vi "Test Filt.vi"() -> ()   [LabVIEW 2024, in "Spectrum Recorder too.lvclass"]
uses:
  Spectrum Recorder too.lvclass
  NHMFL_Core/Libraries/Red Pitaya/RP Core/Red Pitaya Transceiver Driver/Red Pitaya Transceiver Driver.lvclass
  Spectrum Recorder too.lvclass/Spectrum Recorder too.ctl
  NHMFL_Core/Libraries/Red Pitaya/RP Core/RP Transceiver/RP Transceiver.lvclass
  NHMFL_Core/Libraries/Instruments/Instrument Driver/Instrument Driver.lvclass
  NHMFL_Core/Libraries/Instruments/Instrument Driver/Worker State.ctl
  NHMFL_Core/Libraries/Red Pitaya/RP Core/Red Pitaya Transceiver Driver/Spectrum Configuration.ctl
panel:
  out "Status response":u32=1 format="0x%x (%d)"
  out "Waveform Graph":i32[][](graph)
  in  "N point out":i32=16384 format="0x%x (%d)"
  out "Pre -data out 2":i32[](array[numeric])
  out "Pre-data out":i32[](array[numeric])
  out "Points in buffer init":i32
  out "y counter init":u32=1 format="0x%x (%d)"
  out "f counter init":u32=1 format="0x%x (%d)"
  in  "Counters":i32[][](array[numeric])
  in  "Pre-trigger samples":u64
  in  "Post-trigger samples":u64=33554432 format="%.0f (x%x)"
  out "y counter 2":u32=2999 format="0x%x (%d)"
  out "Points in buffer 2":i32=3000
  out "f counter 2":u32=2998 format="0x%x (%d)"
  out "Points in buffer":i32=3003
  out "f counter":u32=3001 format="0x%x (%d)"
  out "y counter":u32=3002 format="0x%x (%d)"
  in  "milliseconds to wait":u32=5000
  out "size(s)":i32=3003
  out "Y":i32[](array[numeric])
  out "X":i32[](array[numeric])
  out "F":dbl[](array[numeric]) format="%_6p"
  out "Sweep duration":dbl=0.786694144 format="%#_gs"
  in  "Configuration":T1={"Start frequency"=500000.0, "End frequency"=2000000.0, "Coarse step"=10000.0, "Step duration"=6.5536e-05, "Red Pitaya address"="192.168.1.120", "Open plot \non start"=TRUE, "Regions width"=2000.0, "Fine step"=10.0, "Pause between scans"=1.0, "Clear rgs on start"=FALSE, "Output amplitude"=1.0, "Append measurements"=[], "Full scan period"=nan, "Full start"=500000.0, "Full end"=2000000.0, "Full step"=100.0} {"Full step" format="%#_6pHz"; "Full end" format="%#_6pHz"; "Full start" format="%#_6pHz"; "Full scan period" format="%#_6fs"; "Output amplitude" min=0.0 max=1.0 step=0.1 format="%#_6pV"; "Pause between scans" format="%#_6ps"; "Fine step" min=0.001 format="%#_6pHz"; "Regions width" format="%#_6pHz"; "Step duration" format="%#_6ps"; "Coarse step" format="%#_6pHz"; "End frequency" format="%#_6pHz"; "Start frequency" format="%#_6pHz"}
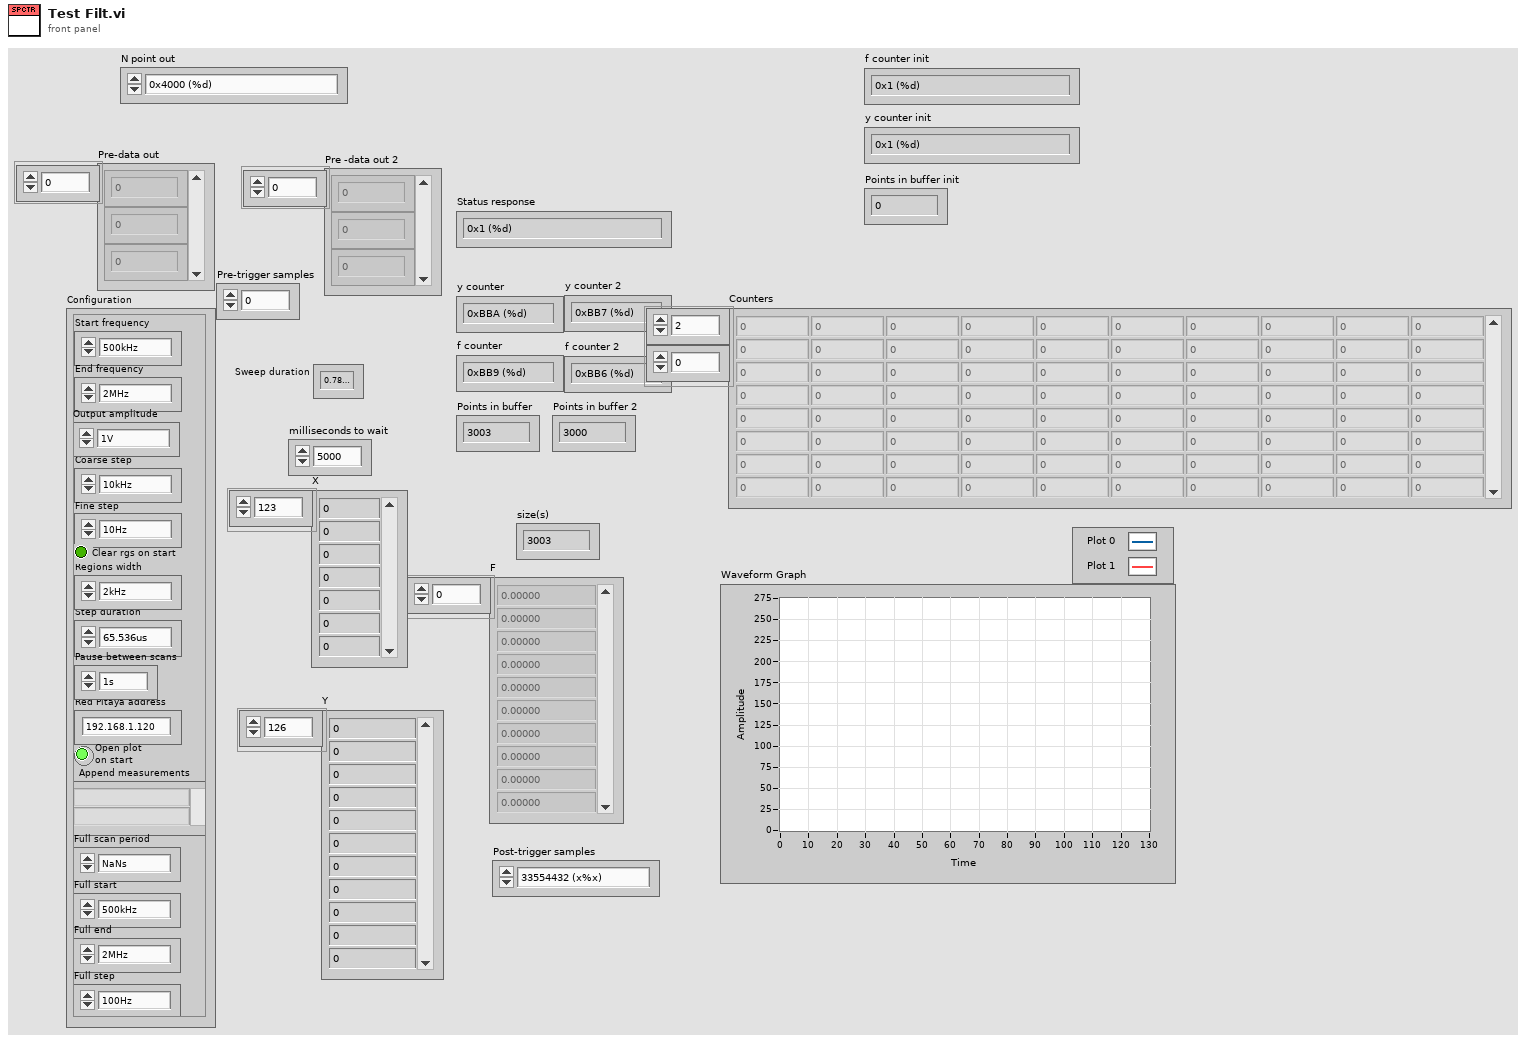
[diagram p1: front panel]
types:
  T1 = typedef "Spectrum Configuration.ctl" = cluster{"Start frequency":dbl, "End frequency":dbl, "Coarse step":dbl, "Step duration":dbl, "Red Pitaya address":string, "Open plot \non start":bool, "Regions width":dbl, "Fine step":dbl, "Pause between scans":dbl, "Clear rgs on start":bool, "Output amplitude":dbl, "Append measurements":string[], "Full scan period":dbl, "Full start":dbl, "Full end":dbl, "Full step":dbl}
  T2 = typedef "Worker State.ctl" = enum16{"Idle", "Starting", "Working", "Stopping"}
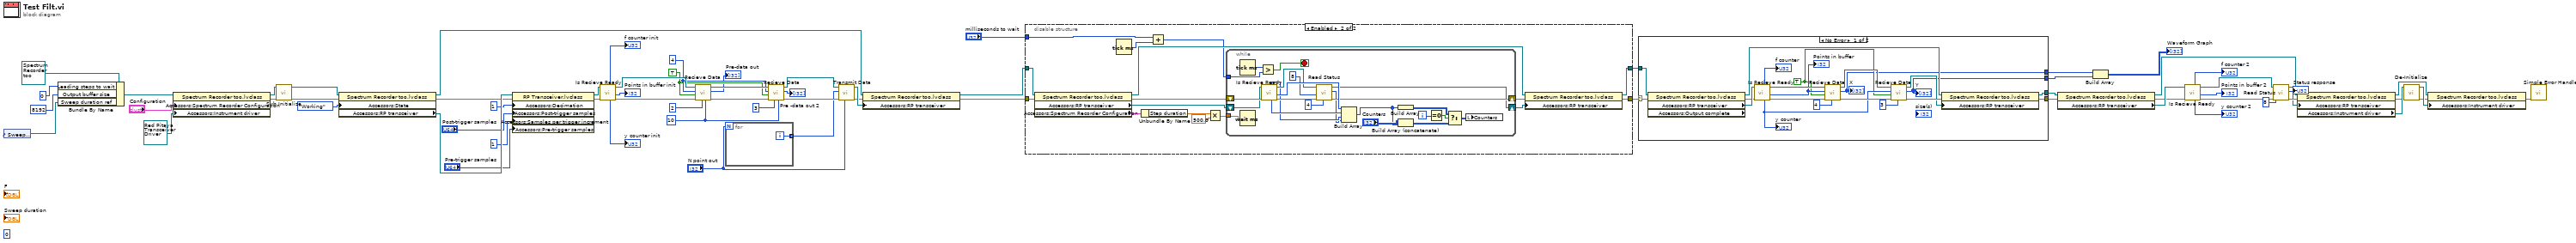
[diagram p0: block diagram]
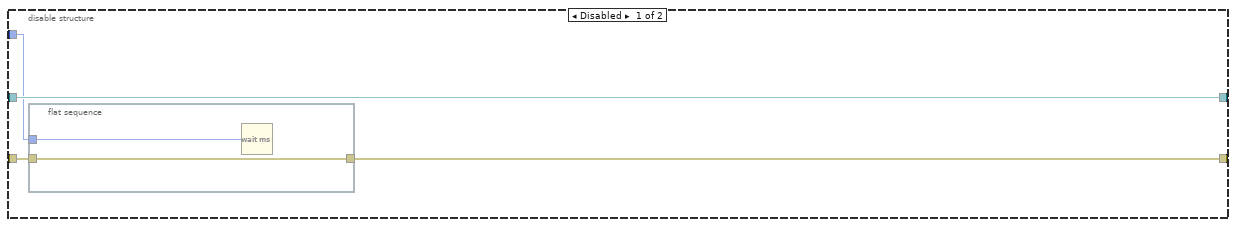
[diagram p2: hidden frame]
diagram:
  w22 = 10 ("timeout ms (25000)")
  w25 = u32 4 ("Points to read")
  w24 = TRUE ("Force read")
  (unwired) i16 0
  n1 = control-ref of="Sweep duration"() -> (w62:refnum<vi>)
  n2 = Bundle By Name(cluster=refnum<class "Spectrum Recorder too.lvclass"> refnum ("Spectrum Recorder too.lvclass"), "Leading steps to wait"=0, "Output buffer size"=8192, "Sweep duration ref"=w62) -> (w63:refnum<class "Spectrum Recorder too.lvclass">)
  n3 = property class="Spectrum Recorder too.lvclass"(reference=w63, "Accessors:Spectrum Recorder Configuration"="Configuration", "Accessors:Instrument driver"=refnum<class "Red Pitaya Transceiver Driver.lvclass"> refnum ("Red Pitaya Transceiver Driver.lvclass")) -> (reference out=w67:refnum<class "Spectrum Recorder too.lvclass">, error out=w65:errorcluster)  [unwired: 1 in]
  n4 = call-dynamic "Sub Initialize.vi"("error in (no error)"=w65, "Spectrum Recorder in"=w67) -> ("error out"=w66:errorcluster, "Spectrum Recorder out"=w58:refnum<class "Spectrum Recorder too.lvclass">)  [unwired: 7 in, 1 out]
  n5 = property class="Spectrum Recorder too.lvclass"(reference=w58, error in=w66, "Accessors:State"=Worker_State."Working" ("State")) -> (reference out=w31:refnum<class "Spectrum Recorder too.lvclass">, error out=w49:errorcluster, "Accessors:RP transceiver"=w52:refnum<class "RP Transceiver.lvclass">)
  n6 = property class="RP Transceiver.lvclass"(reference=w52, error in=w49, "Accessors:Decimation"=1 ("Decimation"), "Accessors:Post-trigger samples"="Post-trigger samples", "Accessors:Samples per trigger increment "=1 ("Samples per trigger increment"), "Accessors:Pre-trigger samples"="Pre-trigger samples") -> (reference out=w19:refnum<class "RP Transceiver.lvclass">, error out=w18:errorcluster)
  n7 = call-dynamic "Is Recieve Ready.vi"("error in (no error)"=w18, "RP Instrument in"=w19) -> ("error out"=w26:errorcluster, "Points in buffer"=→"Points in buffer init":u32, "RP Instrument out"=w29:refnum<class "RP Transceiver.lvclass">, "y counter"=→"y counter init":u32, "f counter"=→"f counter init":u32)  [unwired: 4 in, 1 out]
  n8 = call-dynamic "Recieve Data.vi"("timeout ms (25000)"=w22, "hub port"=u64 2, "error in (no error)"=w26, "Force read"=w24, "Points to read"=w25, "RP Instrument in"=w29) -> ("error out"=w27:errorcluster, "Data out"=→"Pre-data out":i32[], "RP Instrument out"=w28:refnum<class "RP Transceiver.lvclass">)  [unwired: 3 in]
  n9 = for {
    N: "N point out" -> [_]
    tunnel: [w70] -> w13 mode=indexing
    i -> [w70]
  }
  n10 = call-dynamic "Recieve Data.vi"("timeout ms (25000)"=w22, "hub port"=u64 3, "error in (no error)"=w27, "Force read"=w24, "Points to read"=w25, "RP Instrument in"=w28) -> ("error out"=w15:errorcluster, "Data out"=→"Pre -data out 2":i32[], "RP Instrument out"=w17:refnum<class "RP Transceiver.lvclass">)  [unwired: 3 in]
  n11 = call-dynamic "Transmit Data.vi"("Buffer size"="N point out", "error in (no error)"=w15, "Data"=w13, "RP Instrument in"=w17) -> ("error out"=w14:errorcluster, "RP Instrument out"=w16:refnum<class "RP Transceiver.lvclass">)  [unwired: 6 in]
  n12 = property class="Spectrum Recorder too.lvclass"(reference=w31, error in=w14, "Accessors:RP transceiver"=w16) -> (reference out=w42:refnum<class "Spectrum Recorder too.lvclass">, error out=w56:errorcluster)
  n13 = disable-structure shown="Enabled" {
    disable-tunnel: w56 -> [w74 w92]
    disable-tunnel: [w73 w88] -> w55
    disable-tunnel: w42 -> [w72 w85]
    disable-tunnel: [w72 w87] -> w41
    disable-tunnel: "milliseconds to wait" -> [w71 w78]
    frame Disabled {
      n14 = flat-sequence {
        tunnel: w74 -> [w76]
        tunnel: [w76] -> w73
        tunnel: w71 -> [w75]
        frame #0 {
          n15 = Wait (ms)(milliseconds to wait=w75) -> ()  [unwired: 1 out]
        }
      }
    }
    frame Enabled {
      n16 = property class="Spectrum Recorder too.lvclass"(reference=w85, error in=w92) -> (reference out=w86:refnum<class "Spectrum Recorder too.lvclass">, error out=w84:errorcluster, "Accessors:RP transceiver"=w91:refnum<class "RP Transceiver.lvclass">, "Accessors:Spectrum Recorder Configuration"=w83:T1)
      n17 = Tick Count (ms)() -> (millisecond timer value=w79:u32)
      n18 = Unbundle By Name(w83) -> ("Step duration"=w82:dbl)
      n19 = Add(x=w78, y=w79) -> (x+y=w77:u32)
      n20 = Multiply(x=w82, y=500.0) -> (x*y=w80:dbl)
      n21 = while {
        shift-right: [w97] -> w90
        shift-left: w84 -> [w115]
        shift-right: [w96] -> w89
        shift-left: w91 -> [w114]
        tunnel: w80 -> [w113]
        tunnel: w77 -> [w101]
        i -> [w111]
        stop <- w112 stop-if-true
        n22 = Tick Count (ms)() -> (millisecond timer value=w102:u32)
        n23 = Wait (ms)(milliseconds to wait=w113) -> ()  [unwired: 1 out]
        n24 = Greater?(x=w102, y=w101) -> (0:w112:bool)
        n25 = call-dynamic "Is Recieve Ready.vi"("error in (no error)"=w115, "RP Instrument in"=w114) -> ("error out"=w99:errorcluster, "Points in buffer"=w110:u32, "RP Instrument out"=w100:refnum<class "RP Transceiver.lvclass">, "y counter"=w109:u32, "f counter"=w94:u32)  [unwired: 4 in, 1 out]
        n26 = call-dynamic "Read Status.vi"("bytes to read"=4, "error in (no error)"=w99, "Status offset"=u64 8, "RP Instrument in"=w100) -> ("error out"=w97:errorcluster, "Status response"=w93:u32, "RP Instrument out"=w96:refnum<class "RP Transceiver.lvclass">)  [unwired: 5 in]
        n27 = Build Array(w110, w109, w94, w93) -> (w105:u32[])
        n28 = Build Array(w105) -> (w107:u32[][])
        n29 = Build Array (concatenate)("Counters", w105) -> (w104:u32[][])
        n30 = Equal To 0?(x=w111) -> (x = 0?=w108:bool)
        n31 = Select(t=w107, s=w108, f=w104) -> (s? t:f=w103:u32[][])
        n32 = local write "Counters"(w103) -> ()
      }
      n33 = property class="Spectrum Recorder too.lvclass"(reference=w86, error in=w90, "Accessors:RP transceiver"=w89) -> (reference out=w87:refnum<class "Spectrum Recorder too.lvclass">, error out=w88:errorcluster)
    }
  }
  n34 = case shown="No Error" w55 {
    selector: w55 -> [w135 w137]
    tunnel: [w136 w137] -> w48
    tunnel: [w130 w138] -> w33
    tunnel: w41 -> [w134 w138]
    tunnel: [w117 _] -> w11
    tunnel: [w116 _] -> w10
    frame No Error {
      w118 = TRUE ("Force read")
      n35 = property class="Spectrum Recorder too.lvclass" props=["Accessors:RP transceiver", "Accessors:Output complete"](reference=w134, error in=w135) -> (reference out=w131:refnum<class "Spectrum Recorder too.lvclass">, error out=w132:errorcluster, "Accessors:RP transceiver"=w133:refnum<class "RP Transceiver.lvclass">)  [unwired: 1 out]
      n36 = call-dynamic "Is Recieve Ready.vi"("error in (no error)"=w132, "RP Instrument in"=w133) -> ("error out"=w125:errorcluster, "Points in buffer"=w121:u32, "RP Instrument out"=w124:refnum<class "RP Transceiver.lvclass">, "y counter"=w120:u32, "f counter"=→"f counter":u32)  [unwired: 4 in, 1 out]
      "y counter" <- w120
      "Points in buffer" <- w121
      n37 = call-dynamic "Recieve Data.vi"("hub port"=u64 4, "error in (no error)"=w125, "Force read"=w118, "Points to read"=w121, "RP Instrument in"=w124) -> ("error out"=w127:errorcluster, "Data out"=w117:i32[], "RP Instrument out"=w126:refnum<class "RP Transceiver.lvclass">)  [unwired: 4 in]
      "X" <- w117
      n38 = call-dynamic "Recieve Data.vi"("hub port"=u64 3, "error in (no error)"=w127, "Force read"=w118, "Points to read"=w120, "RP Instrument in"=w126) -> ("error out"=w123:errorcluster, "Data out"=w116:i32[], "RP Instrument out"=w122:refnum<class "RP Transceiver.lvclass">)  [unwired: 4 in]
      "Y" <- w116
      n39 = property class="Spectrum Recorder too.lvclass"(reference=w131, error in=w123, "Accessors:RP transceiver"=w122) -> (reference out=w130:refnum<class "Spectrum Recorder too.lvclass">, error out=w136:errorcluster)
    }
    frame Error {
    }
  }
  n40 = property class="Spectrum Recorder too.lvclass"(reference=w33, error in=w48) -> (reference out=w32:refnum<class "Spectrum Recorder too.lvclass">, error out=w7:errorcluster, "Accessors:RP transceiver"=w8:refnum<class "RP Transceiver.lvclass">)
  n41 = Build Array(w11, w10) -> (→"Waveform Graph":i32[][])
  n42 = call-dynamic "Is Recieve Ready.vi"("error in (no error)"=w7, "RP Instrument in"=w8) -> ("error out"=w5:errorcluster, "Points in buffer"=→"Points in buffer 2":u32, "RP Instrument out"=w6:refnum<class "RP Transceiver.lvclass">, "y counter"=→"y counter 2":u32, "f counter"=→"f counter 2":u32)  [unwired: 4 in, 1 out]
  n43 = call-dynamic "Read Status.vi"("error in (no error)"=w5, "Status offset"=u64 8, "RP Instrument in"=w6) -> ("error out"=w4:errorcluster, "Status response"=→"Status response":u32, "RP Instrument out"=w3:refnum<class "RP Transceiver.lvclass">)  [unwired: 6 in]
  n44 = property class="Spectrum Recorder too.lvclass"(reference=w32, error in=w4, "Accessors:RP transceiver"=w3) -> (reference out=w44:refnum<class "Spectrum Recorder too.lvclass">, error out=w43:errorcluster, "Accessors:Instrument driver"=w45:refnum<class "Instrument Driver.lvclass">)
  n45 = call-dynamic "De-Initialize.vi"("error in (no error)"=w43, "Instrument Driver in"=w45) -> ("error out"=w60:errorcluster, "Instrument Driver out"=w61:refnum<class "Instrument Driver.lvclass">)  [unwired: 8 in]
  n46 = property class="Spectrum Recorder too.lvclass"(reference=w44, error in=w60, "Accessors:Instrument driver"=w61) -> (error out=w59:errorcluster)  [unwired: 1 out]
  n47 = call <vilib>:"Simple Error Handler.vi"("error in (no error)"=w59) -> ()  [unwired: 4 in, 5 out]
